vi "set Displacement.vi"(10 "Point":T1, 11 "Motion in":refnum<class "Motion.lvclass">) -> (3 "Motion out":refnum<class "Motion.lvclass">)   [LabVIEW 2015, in "Motion.lvclass"]
uses:
  Motion.lvclass
  LabSDL2/Source/Libraries/SDL2 Utility/Point (I32).ctl
  Motion.lvclass/Motion.ctl
  Vector 2D/Vector 2D.lvclass/Vector 2D.ctl
  Vector 2D/Vector 2D.lvclass
  LabSDL2/Source/Libraries/SDL2 Utility/SDL2 Utility.lvlib
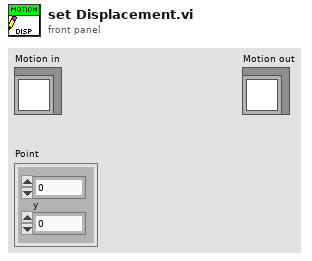
[diagram p1: front panel]
types:
  T1 = typedef "SDL2 Utility.lvlib/Point (I32).ctl" = cluster{"x":i32, "y":i32}
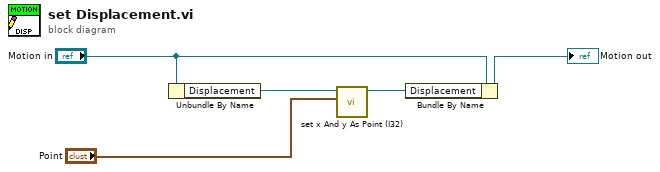
[diagram p0: block diagram]
diagram:
  n1 = Unbundle By Name("Motion in") -> ("Displacement"=w3:refnum<class "Vector 2D.lvclass">)
  n2 = call "set x And y As Point (I32).vi"("Point"="Point", "Vector 2D in"=w3) -> ("Vector 2D out"=w2:refnum<class "Vector 2D.lvclass">)  [unwired: 9 in]
  n3 = Bundle By Name(cluster="Motion in", "Displacement"=w2) -> (→"Motion out":refnum<class "Motion.lvclass">)
